vi "Check If it Has Run.vi"(8 "error in (no error)":errorcluster, 10 "Application_Name(\"\")":string, 11 "Admin_Actor in":refnum<class "Admin_Actor.lvclass">) -> (0 "error out":errorcluster, 2 "Has(False)":bool, 3 "Admin_Actor out":refnum<class "Admin_Actor.lvclass">)   [LabVIEW 2015]
uses:
  Admin_Actor.lvclass
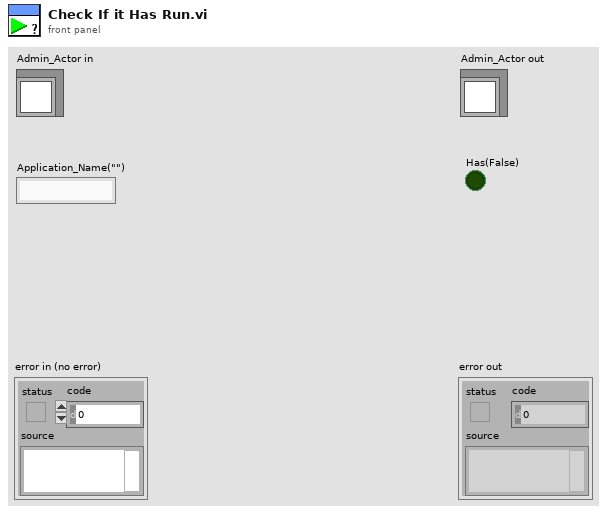
[diagram p1: front panel]
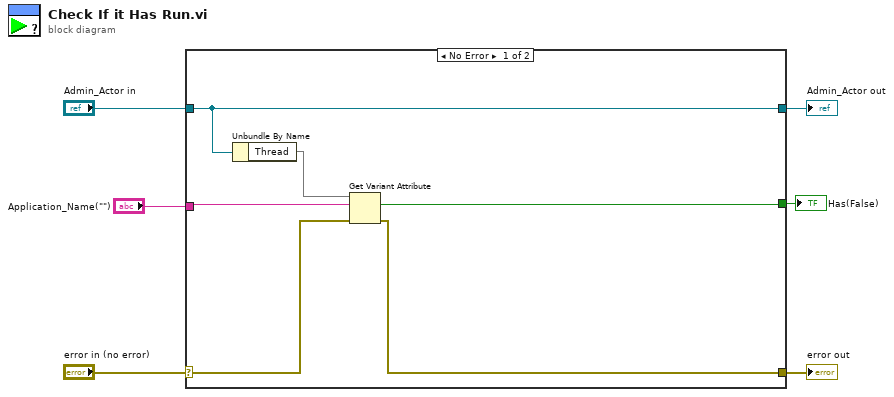
[diagram p0: block diagram]
diagram:
  n1 = case shown="No Error" "error in (no error)" {
    selector: "error in (no error)" -> [w9 w14]
    tunnel: [w8 w14] -> w5
    tunnel: [w12 w13] -> w3
    tunnel: "Admin_Actor in" -> [w12 w13]
    tunnel: "Application_Name(\"\")" -> [w10 _]
    tunnel: [w7 _] -> w1
    frame No Error {
      n2 = Unbundle By Name(w12) -> ("Thread"=w11)
      n3 = Get Variant Attribute(Variant=w11, name=w10, error in=w9) -> (found=w7:bool, error out=w8:errorcluster)  [unwired: 1 in, 2 out]
    }
    frame Error {
    }
  }
  "error out" <- w5
  "Admin_Actor out" <- w3
  "Has(False)" <- w1
